vi "Handle Value Change.vi"(5 "VolatusAPI":refnum<class "VolatusAPI.lvclass">, 7 "CtlRef":refnum<vi>, 8 "error in (no error)":errorcluster, 9 "NewVal":variant, 10 "OldVal":variant, 11 "2WayValve in":refnum<class "2WayValve.lvclass">) -> (0 "error out":errorcluster, 3 "2WayValve out":refnum<class "2WayValve.lvclass">)   [LabVIEW 2020, in "VolatusGUIElements.lvlib" / "2WayValve.lvclass"]
uses:
  2WayValve.lvclass
  Volatus/VolatusAPI/VolatusAPI.lvclass
  2WayValve.lvclass/2WayValve.ctl
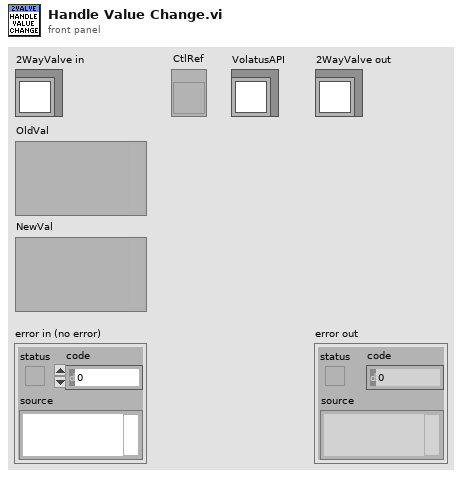
[diagram p1: front panel]
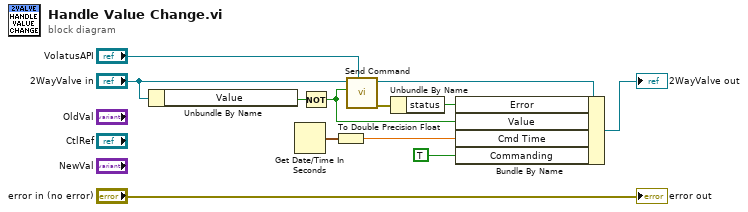
[diagram p0: block diagram]
diagram:
  n1 = Unbundle By Name("2WayValve in") -> ("Value"=w5:bool)
  n2 = Get Date/Time In Seconds() -> (seconds since 1Jan1904=w3:timestamp)
  n3 = Not(x=w5) -> (.not. x?=w4:bool)
  n4 = To Double Precision Float(number=w3) -> (double precision float=w2:dbl)
  n5 = call "Send Command.vi"("VolatusAPI"="VolatusAPI", "Value"=w4, "2WayValve in"="2WayValve in") -> ("error out"=w9:errorcluster, "2WayValve out"=w11:refnum<class "2WayValve.lvclass">)  [unwired: 7 in]
  n6 = Unbundle By Name(w9) -> ("status"=w8:bool)
  n7 = Bundle By Name(cluster=w11, "Error"=w8, "Value"=w4, "Cmd Time"=w2, "Commanding"=TRUE) -> (→"2WayValve out":refnum<class "2WayValve.lvclass">)
  "error out" <- "error in (no error)"
